vi "Exercises FM Demodulation.vi"(8 "错误输入":errorcluster, 10 "重采样率":dbl, 11 "接收信号":waveform(cdb)) -> (0 "错误输出":errorcluster, 2 "重采样后信号":waveform(dbl)(graph), 3 "解调后信号":waveform(dbl)(graph))   [LabVIEW 2015]
uses:
  <vilib>/measure/NI_MAPro.lvlib
  <vilib>/measure/maresamp.llb/Resample Waveform (continuous).vi
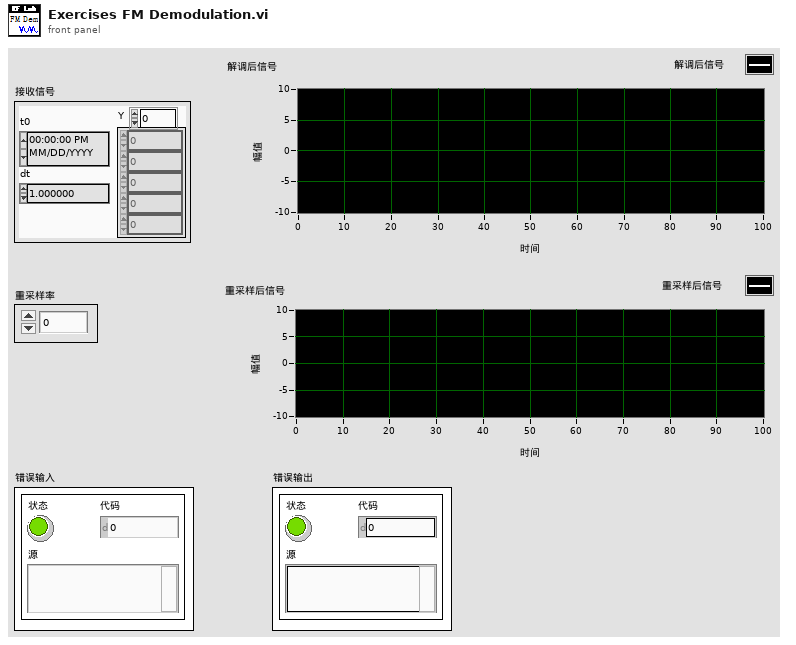
[diagram p1: front panel]
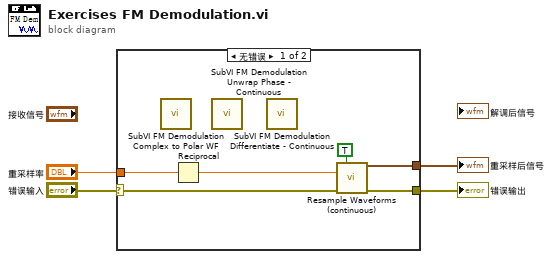
[diagram p0: block diagram]
diagram:
  n1 = case shown="无错误" "错误输入" {
    selector: "错误输入" -> [w5 w11]
    tunnel: "重采样率" -> [w10 _]
    tunnel: [w9 _] -> w3
    tunnel: [w8 w11] -> w2
    frame No Error {
      n2 = call "SubVI FM Demodulation Complex to Polar WF.vi"() -> ()  [unwired: 1 in, 2 out]
      n3 = Reciprocal(x=w10) -> (1/x=w7:dbl)
      n4 = call "SubVI FM Demodulation Unwrap Phase - Continuous.vi"() -> ()  [unwired: 2 in, 1 out]
      n5 = call "SubVI FM Demodulation Differentiate - Continuous.vi"() -> ()  [unwired: 3 in, 1 out]
      n6 = call-poly <vilib>:"Resample Waveforms (continuous).vi"("reset"=TRUE, "dt"=w7, "error in (no error)"=w5) -> ("resampled waveform out"=w9:waveform(dbl), "error out"=w8:errorcluster)  [unwired: 8 in, 3 out]
    }
    frame Error {
    }
  }
  "重采样后信号" <- w3
  "错误输出" <- w2
